vi "Init Values.vi"(8 "error in (no error)":errorcluster, 11 "ValveControlModule in":refnum<class "DigitalControlModule.lvclass">) -> (0 "error out":errorcluster, 3 "ValveControlModule out":refnum<class "DigitalControlModule.lvclass">)   [LabVIEW 2020, in "VolatusControl.lvlib" / "DigitalControlModule.lvclass"]
uses:
  DigitalControlModule.lvclass
  C:/dev/lv20CE/relink/lv-volatus/Volatus/Module/Module.lvclass
  Volatus/Module/Module.lvclass/Module.ctl
  DigitalControlModule.lvclass/DigitalControlModule.ctl
  VolatusConfig/VolatusConfigElement/VolatusConfigElement.lvclass/VolatusConfigElement.ctl
  Volatus/Module/Config.vi
  VolatusConfig/VolatusConfigElement/Element.vi
  VolatusConfig/Task/Task.lvclass
  C:/dev/lv20CE/relink/lv-volatus/VolatusConfig/VolatusConfigElement/VolatusConfigElement.lvclass
  lv-vecto/Vecto/Group/Group.lvclass
  C:/dev/lv20CE/relink/lv-vecto/Vecto/GroupAbstract/GroupAbstract.lvclass
  lv-cdm/CDM-Config/Config Element/Owner.vi
  lv-cdm/CDM-Config/Config Manager/Lookup Descendant.vi
  Volatus/Module/Module.lvclass
  VolatusConfig/VolatusConfigElement/VolatusConfigElement.lvclass
  lv-cdm/CDM-Config/Config Filter/Config Lookup.lvclass
  lv-cdm/CDM-Config/Config Element/Config Element.lvclass
  lv-vecto/Vecto/GroupAbstract/GroupAbstract.lvclass
  C:/dev/lv20CE/relink/lv-volatus/VolatusConfig/Task/Task.lvclass
  C:/dev/lv20CE/relink/lv-vecto/Vecto/Group/Group.lvclass
  C:/dev/lv20CE/relink/lv-volatus/VolatusControl/ValveControlModule/DigitalControlModule.lvclass
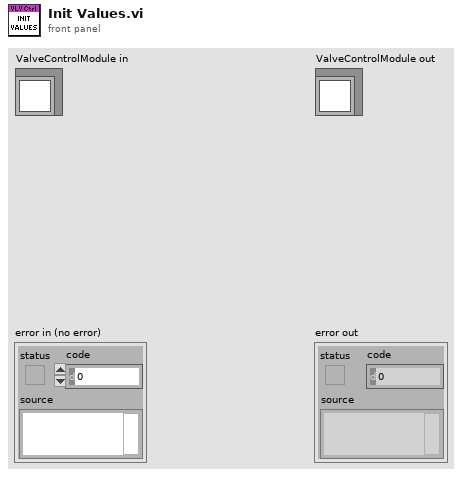
[diagram p1: front panel]
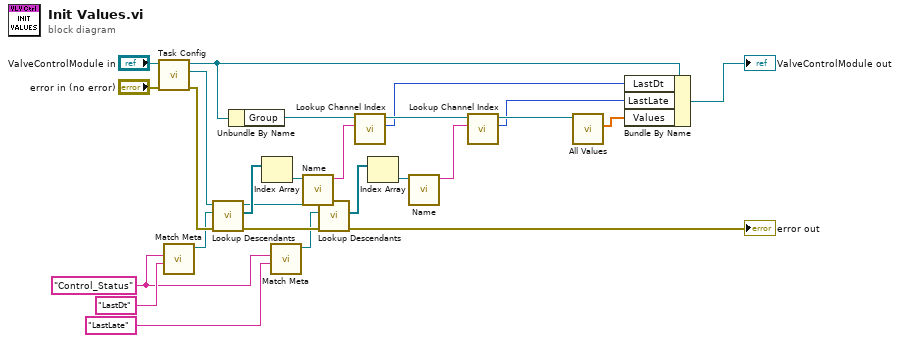
[diagram p0: block diagram]
diagram:
  w2 = "Control_Status" ("Name")
  n1 = call "Task Config.vi"("error in (no error)"="error in (no error)", "Module in"="ValveControlModule in") -> ("error out"=w26:errorcluster, "Task Config"=w22:refnum<class "Task.lvclass">, "Module out"=w10:refnum<class "DigitalControlModule.lvclass">)  [unwired: 7 in]
  n2 = call "Match Meta.vi"("Value (Any)"="LastDt" ("Name"), "Name"=w2) -> ("Config Lookup out"=w19:refnum<class "Config Lookup.lvclass">)  [unwired: 8 in, 1 out]
  n3 = call "Lookup Descendants.vi"("error in (no error)"=w26, "Lookup"=w19, "VolatusConfigElement in"=w22) -> ("error out"=w13:errorcluster, "Descendants"=w21:refnum<class "Config Element.lvclass">[], "VolatusConfigElement out"=w12:refnum<class "Task.lvclass">)  [unwired: 6 in]
  n4 = Unbundle By Name(w10) -> ("Group"=w25:refnum<class "Group.lvclass">)
  n5 = Index Array(array=w21) -> (element=w16:refnum<class "Config Element.lvclass">)  [unwired: 1 in]
  n6 = call "Match Meta.vi"("Value (Any)"="LastLate" ("Name"), "Name"=w2) -> ("Config Lookup out"=w3:refnum<class "Config Lookup.lvclass">)  [unwired: 8 in, 1 out]
  n7 = call "Name.vi"("Config Element in"=w16) -> ("Name"=w7:string)  [unwired: 9 in, 1 out]
  n8 = call "Lookup Descendants.vi"("error in (no error)"=w13, "Lookup"=w3, "VolatusConfigElement in"=w12) -> ("error out"=→"error out":errorcluster, "Descendants"=w14:refnum<class "Config Element.lvclass">[])  [unwired: 6 in, 1 out]
  n9 = call "Lookup Channel Index.vi"("Channel Name"=w7, "GroupAbstract in"=w25) -> ("Index"=w4:i32, "GroupAbstract out"=w9:refnum<class "Group.lvclass">)  [unwired: 7 in, 1 out]
  n10 = Index Array(array=w14) -> (element=w15:refnum<class "Config Element.lvclass">)  [unwired: 1 in]
  n11 = call "Name.vi"("Config Element in"=w15) -> ("Name"=w6:string)  [unwired: 9 in, 1 out]
  n12 = call "Lookup Channel Index.vi"("Channel Name"=w6, "GroupAbstract in"=w9) -> ("Index"=w5:i32, "GroupAbstract out"=w8:refnum<class "Group.lvclass">)  [unwired: 7 in, 1 out]
  n13 = call "All Values.vi"("Group in"=w8) -> ("Scaled"=w23:dbl[])  [unwired: 6 in, 4 out]
  n14 = Bundle By Name(cluster=w10, "LastDt"=w4, "LastLate"=w5, "Values"=w23) -> (→"ValveControlModule out":refnum<class "DigitalControlModule.lvclass">)
